vi "arrayvariant.vi"(1 "Array In":variant[](array[variant]), 2 "String To Append":string, 3 "Base":dbl format="%.2f") -> (0 "Array Out":variant[](array[variant]))   [LabVIEW 2011]
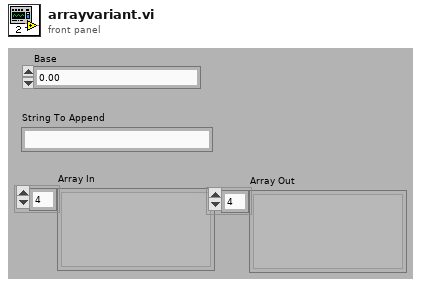
[diagram p1: front panel]
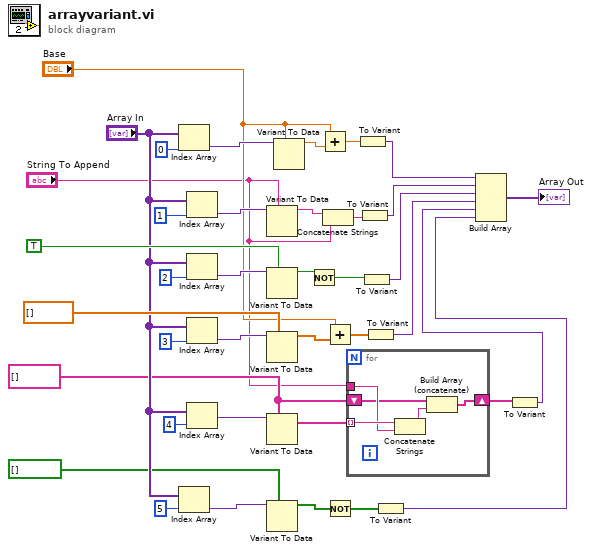
[diagram p0: block diagram]
diagram:
  w9 = string[] []
  n1 = Index Array(array="Array In", index=0) -> (element=w37:variant)
  n2 = Index Array(array="Array In", index=5) -> (element=w5:variant)
  n3 = Index Array(array="Array In", index=1) -> (element=w31:variant)
  n4 = Index Array(array="Array In", index=2) -> (element=w26:variant)
  n5 = Index Array(array="Array In", index=3) -> (element=w20:variant)
  n6 = Index Array(array="Array In", index=4) -> (element=w11:variant)
  n7 = Variant To Data(type="String To Append", Variant=w31) -> (data=w30:string)  [unwired: 1 in, 1 out]
  n8 = Variant To Data(type=TRUE, Variant=w26) -> (data=w24:bool)  [unwired: 1 in, 1 out]
  n9 = Variant To Data(type=dbl[] [], Variant=w20) -> (data=w18:dbl[])  [unwired: 1 in, 1 out]
  n10 = Variant To Data(type=w9, Variant=w11) -> (data=w10:string[])  [unwired: 1 in, 1 out]
  n11 = Variant To Data(type=bool[] [], Variant=w5) -> (data=w3:bool[])  [unwired: 1 in, 1 out]
  n12 = Variant To Data(type="Base", Variant=w37) -> (data=w36:dbl)  [unwired: 1 in, 1 out]
  n13 = Not(x=w24) -> (.not. x?=w23:bool)
  n14 = Add(x="Base", y=w36) -> (x+y=w35:dbl)
  n15 = Concatenate Strings(w30, "String To Append") -> (w29:string)
  n16 = Add(x="Base", y=w18) -> (x+y=w16:dbl[])
  n17 = Not(x=w3) -> (.not. x?=w2:bool[])
  n18 = for {
    tunnel: w10 -> [w43] mode=indexing
    shift-right: [w39] -> w7
    shift-left: w9 -> [w40]
    tunnel: "String To Append" -> [w42]
    n19 = Concatenate Strings(w43, w42) -> (w41:string)
    n20 = Build Array (concatenate)(w40, w41) -> (w39:string[])
  }
  n21 = To Variant(anything=w35) -> (Variant=w34:variant)
  n22 = To Variant(anything=w29) -> (Variant=w28:variant)
  n23 = To Variant(anything=w23) -> (Variant=w22:variant)
  n24 = To Variant(anything=w16) -> (Variant=w15:variant)
  n25 = To Variant(anything=w2) -> (Variant=w1:variant)
  n26 = To Variant(anything=w7) -> (Variant=w6:variant)
  n27 = Build Array(w34, w28, w22, w15, w6, w1) -> (→"Array Out":variant[])
